vi "Update Processing Metrics.vi"(8 "error in (no error)":errorcluster, 9 "Peak Output":dbl, 10 "System Throughput":dbl, 11 "UI Root in":refnum<class "UI Root.lvclass">) -> (0 "error out":errorcluster, 3 "UI Root out":refnum<class "UI Root.lvclass">)   [LabVIEW 2020, in "UI Root.lvlib" / "UI Root.lvclass"]
uses:
  UI Root.lvclass
  UI Root.lvclass/UI Root.ctl
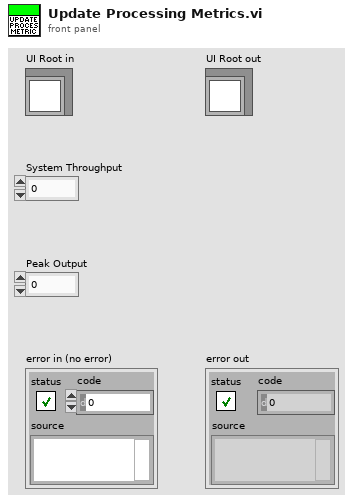
[diagram p1: front panel]
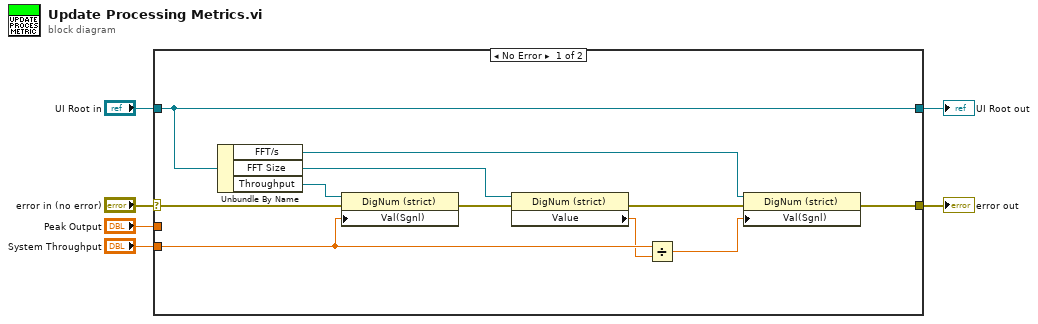
[diagram p0: block diagram]
diagram:
  n1 = case shown="No Error" "error in (no error)" {
    selector: "error in (no error)" -> [w16 w19]
    tunnel: [w9 w19] -> w5
    tunnel: [w17 w18] -> w3
    tunnel: "UI Root in" -> [w17 w18]
    tunnel: "Peak Output" -> [_ _]
    tunnel: "System Throughput" -> [w12 _]
    frame No Error {
      n2 = Unbundle By Name(w17) -> ("FFT/s"=w8:refnum<vi>, "FFT Size"=w13:refnum<vi>, "Throughput"=w15:refnum<vi>)
      n3 = property class="DigNum (strict)"(reference=w15, error in=w16, "Val(Sgnl)"=w12) -> (error out=w14:errorcluster)  [unwired: 1 out]
      n4 = property class="DigNum (strict)"(reference=w13, error in=w14) -> (error out=w10:errorcluster, "Value"=w11:dbl)  [unwired: 1 out]
      n5 = Divide(x=w12, y=w11) -> (x/y=w7:dbl)
      n6 = property class="DigNum (strict)"(reference=w8, error in=w10, "Val(Sgnl)"=w7) -> (error out=w9:errorcluster)  [unwired: 1 out]
    }
    frame Error {
    }
  }
  "error out" <- w5
  "UI Root out" <- w3
